vi "Find VI Target and Path.vi"(10 "Children[]":refnum<vi>[](array[refnum]), 11 "Name":string) -> (2 "Found?":bool, 3 "ThisRef":refnum<vi>)   [LabVIEW 2016]
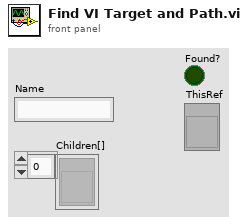
[diagram p1: front panel]
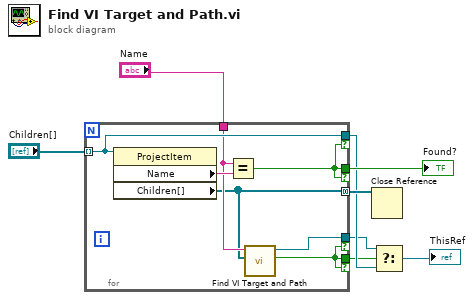
[diagram p0: block diagram]
diagram:
  n1 = for {
    tunnel: "Children[]" -> [w14] mode=indexing
    tunnel: "Name" -> [w12]
    tunnel: [w11] -> w6 mode=concatenating
    tunnel: [w14] -> w4 if=w13
    tunnel: [w13] -> w5 if=w13
    tunnel: [w9] -> w2 if=w9
    tunnel: [w10] -> w1 if=w9
    n2 = property class="ProjectItem"(reference=w14) -> ("Name"=w15:string, "Children[]"=w11:refnum<vi>[])  [unwired: 1 in, 2 out]
    n3 = Equal?(x=w12, y=w15) -> (x = y?=w13:bool)
    n4 = call "Find VI Target and Path.vi"("Children[]"=w11, "Name"=w12) -> ("Found?"=w9:bool, "ThisRef"=w10:refnum<vi>)  [unwired: 8 in]
  }
  "Found?" <- w5
  n5 = Close Reference(reference=w6) -> ()  [unwired: 1 in, 1 out]
  n6 = Select(t=w1, s=w2, f=w4) -> (s? t:f=→"ThisRef":refnum<vi>)
